vi "in plane scan.vi"(6 "invert y":bool, 7 "invert x":bool, 8 "abs(x,y)":bool, 9 "rotate by (degrees)":dbl, 10 "angle (degrees)":dbl, 11 "v total":dbl) -> (0 "v_y string":string, 1 "v_x string":string, 2 "v_y":dbl, 3 "v_x":dbl, 4 "rotated angle":dbl, 5 "rotated rad":dbl)   [LabVIEW 2018]
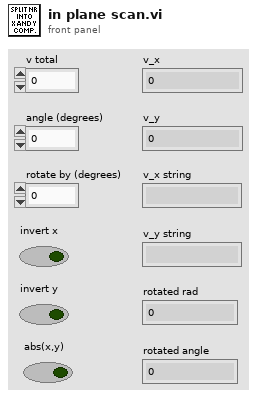
[diagram p1: front panel]
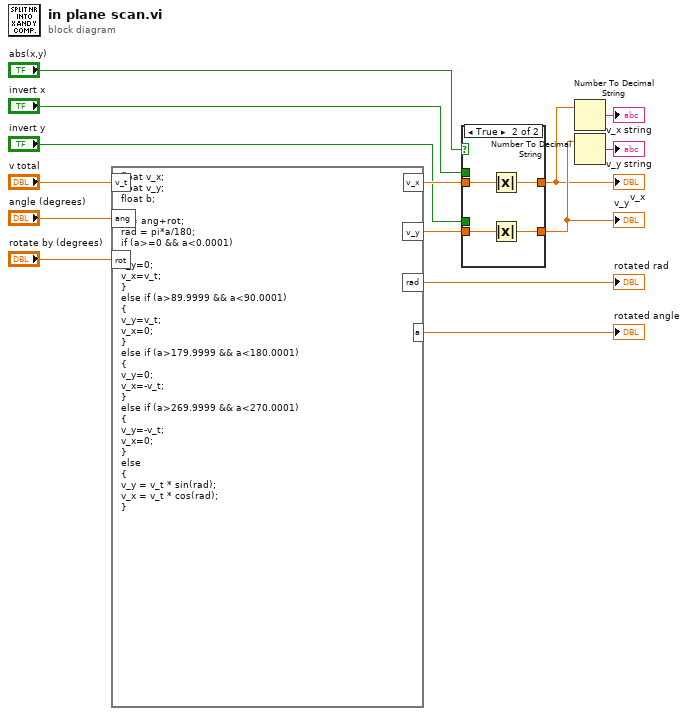
[diagram p0: block diagram]
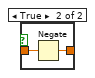
[diagram p3: hidden frame]
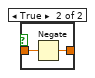
[diagram p4: hidden frame]
diagram:
  n1 = formula code="float v_x;\nfloat v_y;\nfloat b;\n\na = ang+rot;\nrad = pi*a/180;\nif (a>=0 && a<0.0001)\n{\nv_y=0;\nv_x=v_t;\n}\nelse if (a>89.9999 && a<90.0001)\n{\nv_y=v_t;\nv_x=0;\n}\nelse if (a>179.9999 && a<180.0001)\n{\nv_y=0;\nv_x=-v_t;\n}\nelse if (a>269.9999 && a<270.0001)\n{\nv_y=-v_t;\nv_x=0;\n}\nelse\n{\nv_y = v_t * sin(rad);\nv_x = v_t * cos(rad);\n}"("v_t"="v total", "ang"="angle (degrees)", "rot"="rotate by (degrees)") -> ("v_x"=w6:dbl, "v_y"=w4:dbl, "rad"=→"rotated rad":dbl, "a"=→"rotated angle":dbl)
  n2 = case shown="True" "abs(x,y)" {
    tunnel: "invert x" -> [w20 _]
    tunnel: w6 -> [w19 w30]
    tunnel: "invert y" -> [w18 _]
    tunnel: w4 -> [w17 w29]
    tunnel: [w16 w27] -> w3
    tunnel: [w15 w28] -> w2
    frame False {
      n3 = case shown="False" w20 {
        tunnel: w19 -> [w24 w26]
        tunnel: [w24 w25] -> w15
        frame False {
        }
        frame True {
          n4 = Negate(x=w26) -> (-x=w25:dbl)
        }
      }
      n5 = case shown="False" w18 {
        tunnel: w17 -> [w21 w23]
        tunnel: [w21 w22] -> w16
        frame False {
        }
        frame True {
          n6 = Negate(x=w23) -> (-x=w22:dbl)
        }
      }
    }
    frame True {
      n7 = Absolute Value(x=w30) -> (abs(x)=w28:dbl)
      n8 = Absolute Value(x=w29) -> (abs(x)=w27:dbl)
    }
  }
  "v_x" <- w2
  "v_y" <- w3
  n9 = Number To Decimal String(number=w2) -> (decimal integer string=→"v_x string":string)  [unwired: 1 in]
  n10 = Number To Decimal String(number=w3) -> (decimal integer string=→"v_y string":string)  [unwired: 1 in]
